vi "Write iSpkEn.vi"(8 "error in (no error)":errorcluster, 10 "iSpkEn":bool[](array[boolean]), 11 "Set iSpkEn MSG in":refnum<class "Set iSpkEn MSG.lvclass">) -> (0 "error out":errorcluster, 3 "Set iSpkEn MSG out":refnum<class "Set iSpkEn MSG.lvclass">)   [LabVIEW 2014, in "ePAS Library.lvlib" / "Set iSpkEn MSG.lvclass"]
uses:
  Set iSpkEn MSG.lvclass
  Set iSpkEn MSG.lvclass/Set iSpkEn MSG.ctl
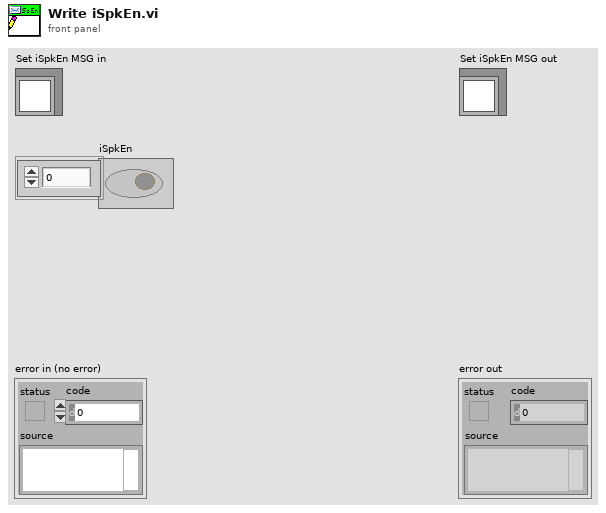
[diagram p1: front panel]
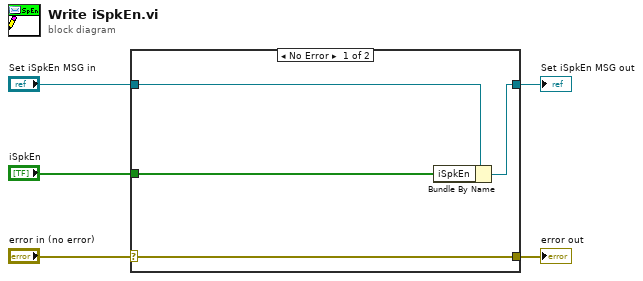
[diagram p0: block diagram]
diagram:
  n1 = case shown="No Error" "error in (no error)" {
    selector: "error in (no error)" -> [w9 w10]
    tunnel: [w9 w10] -> w4
    tunnel: [w7 w11] -> w2
    tunnel: "Set iSpkEn MSG in" -> [w8 w11]
    tunnel: "iSpkEn" -> [w6 _]
    frame No Error {
      n2 = Bundle By Name(cluster=w8, "iSpkEn"=w6) -> (w7:refnum<class "Set iSpkEn MSG.lvclass">)
    }
    frame Error {
    }
  }
  "error out" <- w4
  "Set iSpkEn MSG out" <- w2
